vi "seven_seg_facade.vi"(0 "Data In":T4, 2 "Display State In":T2, 3 "Container State":T3) -> (6 "Data Out":T4, 7 "Display State Out":T2, 8 "Action":T1)   [LabVIEW 2018, in "Seven_seg_disp.xctl"]
uses:
  Seven_seg_disp.xctl
  seven_seg_data.ctl
  <vilib>/_xctls/Container State.ctl
  seven_seg_state.ctl
  <vilib>/_xctls/Action.ctl
  <vilib>/_xctls/XControlSupport.lvlib
panel:
  out "dp":bool
  out "g":bool
  out "f":bool
  out "e":bool
  out "d":bool
  out "c":bool
  out "b":bool
  out "a":bool
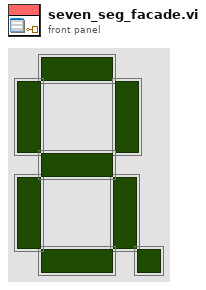
[diagram p1: front panel]
types:
  T1 = typedef "XControlSupport.lvlib/Action.ctl" = cluster{"Data Changed?":bool, "State Changed?":bool, "Action Name":string}
  T2 = typedef "Seven_seg_disp.xctl/seven_seg_state.ctl" = cluster{"Numeric":u8}
  T3 = typedef "XControlSupport.lvlib/Container State.ctl" = cluster{"Indicator?":bool, "Run Mode?":bool, " Refnum":refnum<vi>}
  T4 = typedef "Seven_seg_disp.xctl/seven_seg_data.ctl" = u8
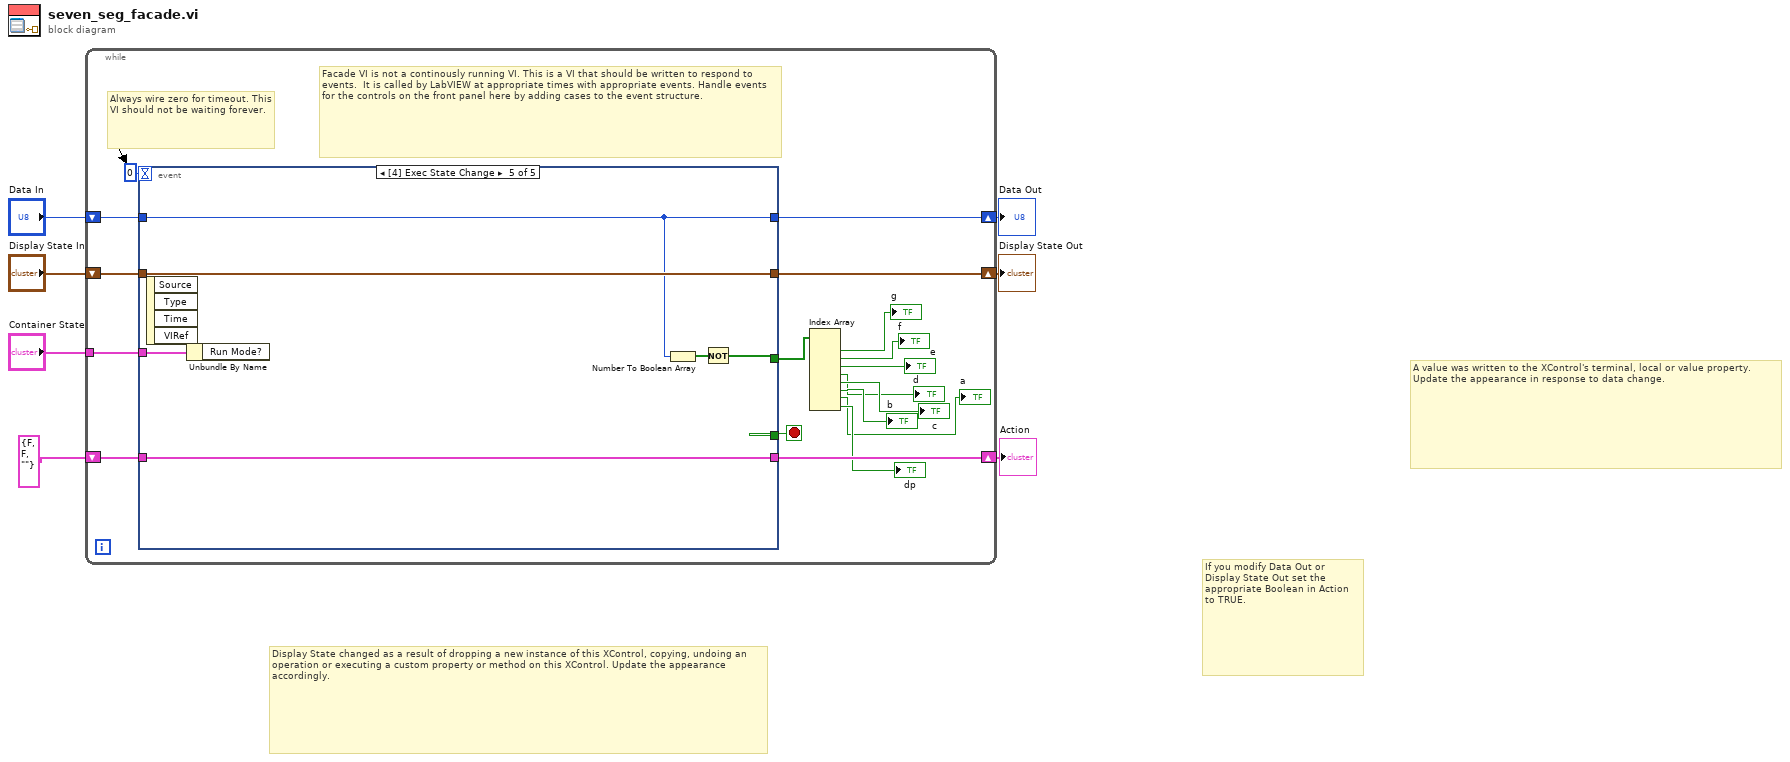
[diagram p0: block diagram]
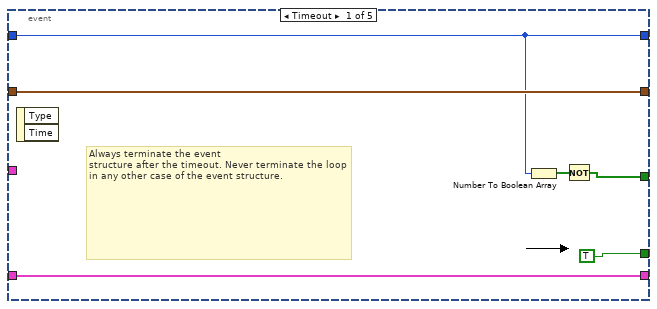
[diagram p2: hidden frame]
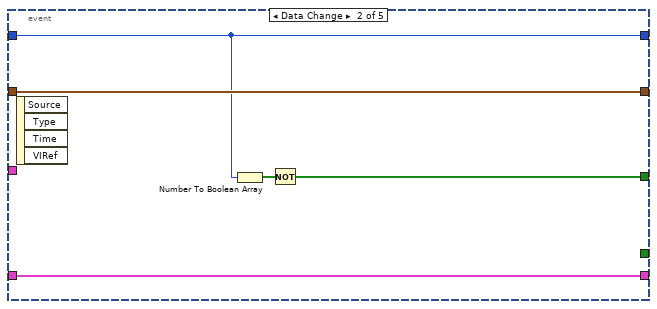
[diagram p3: hidden frame]
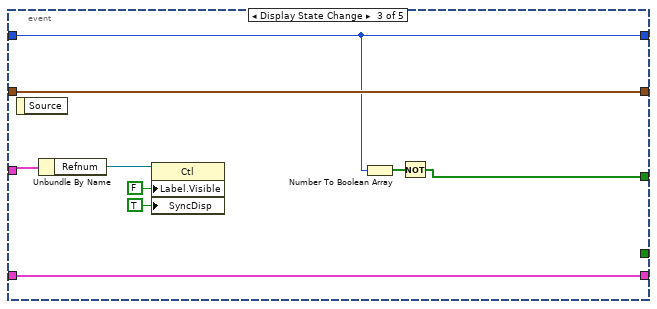
[diagram p4: hidden frame]
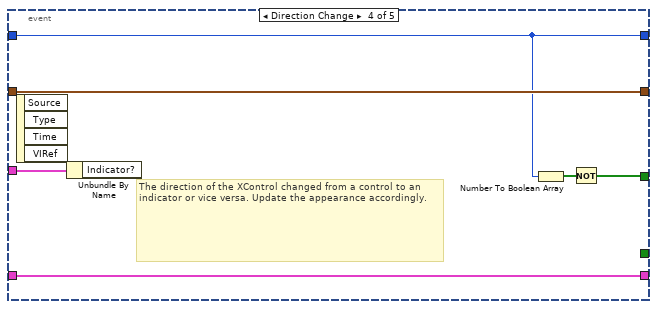
[diagram p5: hidden frame]
diagram:
  # "Display State changed as a result of dropping a new instance of this XControl, copying, undoing an operation or executing a custom property or method on this XControl. Update the appearance accordingly."
  # "A value was written to the XControl's terminal, local or value property.\nUpdate the appearance in response to data change."
  # "If you modify Data Out or\nDisplay State Out set the\nappropriate Boolean in Action\nto TRUE."
  n1 = while {
    shift-right: [w24] -> w4
    shift-left: "Display State In" -> [w25]
    tunnel: "Container State" -> [w21]
    shift-right: [w19] -> w7
    shift-left: "Data In" -> [w20]
    shift-right: [w17] -> w2
    shift-left: T1 {"Data Changed?"=FALSE, "State Changed?"=FALSE, "Action Name"=""} ("Action") -> [w18]
    stop <- w23 stop-if-true
    # "Facade VI is not a continously running VI. This is a VI that should be written to respond to events.  It is called by LabVIEW at appropriate times with appropriate events. Handle events for the controls on the front panel here by adding cases to the event structure."
    # "Always wire zero for timeout. This\nVI should not be waiting forever."
    n2 = event shown="[4] Exec State Change" {
      selector: _ -> [_ _ _ _ _]
      dyn-events: _ -> [_ _ _ _ _]
      timeout: 0 -> [_ _ _ _ _]
      tunnel: w25 -> [w29 w36 w45 w50 w56]
      tunnel: [w29 w36 w45 w50 w56] -> w24
      tunnel: [TRUE _ _ _ _] -> w23
      tunnel: w21 -> [_ _ w43 w51 w57]
      tunnel: w20 -> [w26 w34 w38 w46 w52]
      tunnel: [w26 w34 w38 w46 w52] -> w19
      tunnel: [w30 w35 w44 w49 w55] -> w17
      tunnel: w18 -> [w30 w35 w44 w49 w55]
      tunnel: [w27 w32 w39 w47 w53] -> w8
      event Timeout {
        # "Always terminate the event\nstructure after the timeout. Never terminate the loop in any other case of the event structure."
        n3 = event-data() -> ()  [unwired: 1 in, 2 out]
        n4 = Number To Boolean Array(number=w26) -> (Boolean array=w28:bool[])
        n5 = Not(x=w28) -> (.not. x?=w27:bool[])
      }
      event Data Change {
        n6 = event-data() -> ()  [unwired: 1 in, 4 out]
        n7 = Number To Boolean Array(number=w34) -> (Boolean array=w33:bool[])
        n8 = Not(x=w33) -> (.not. x?=w32:bool[])
      }
      event Display State Change {
        n9 = event-data() -> ()  [unwired: 1 in, 1 out]
        n10 = Unbundle By Name(w43) -> ("Refnum"=w42:refnum<vi>)
        n11 = property class="Ctl"(reference=w42, "Label.Visible"=FALSE, "SyncDisp"=TRUE ("Synchronous Display")) -> ()  [unwired: 1 in, 2 out]
        n12 = Number To Boolean Array(number=w38) -> (Boolean array=w40:bool[])
        n13 = Not(x=w40) -> (.not. x?=w39:bool[])
      }
      event Direction Change {
        # "The direction of the XControl changed from a control to an indicator or vice versa. Update the appearance accordingly."
        n14 = event-data() -> ()  [unwired: 1 in, 4 out]
        n15 = Unbundle By Name(w51) -> ()  [unwired: 1 out]
        n16 = Number To Boolean Array(number=w46) -> (Boolean array=w48:bool[])
        n17 = Not(x=w48) -> (.not. x?=w47:bool[])
      }
      event Exec State Change {
        n18 = event-data() -> ()  [unwired: 1 in, 4 out]
        n19 = Unbundle By Name(w57) -> ()  [unwired: 1 out]
        n20 = Number To Boolean Array(number=w52) -> (Boolean array=w54:bool[])
        n21 = Not(x=w54) -> (.not. x?=w53:bool[])
      }
    }
    n22 = Index Array(array=w8) -> (element #1=→"g":bool, element #2=→"f":bool, element #3=→"e":bool, element #4=→"d":bool, element #5=→"c":bool, element #6=→"b":bool, element #7=→"a":bool, element #8=→"dp":bool)  [unwired: 8 in]
  }
  "Display State Out" <- w4
  "Data Out" <- w7
  "Action" <- w2
